vi "Open.vi"(8 "Error In":errorcluster, 9 "StartupConfiguration":string, 11 "reference in":refnum<class "AppConfigJSON.lvclass">) -> (0 "Error Out":errorcluster, 3 "reference out":refnum<class "AppConfigJSON.lvclass">)   [LabVIEW 2021, in "AppConfigJSON.lvclass"]
uses:
  AppConfigJSON.lvclass
  <vilib>/JDP Science/JSONtext/Config Files/Config File.lvclass/Config File.ctl
  1435ef73-8409-4d57-913a-7b04ec8072c7.vi
  aab25018-df5b-4ee7-aaa7-56694cb3da64.vi
  e6364923-a397-4d7b-ac40-c42afb6024f9.vi
  0d2aa625-af8f-4f9d-94fd-328c4132ffee.vi
  <vilib>/TriekselSoft/TracerLibrary/TracerLibrary/Tracer/protected/SendMessage.vi
  <vilib>/TriekselSoft/TracerLibrary/TracerLibrary/Tracer/protected/Timestamp.vi
  0d2aa625-af8f-4f9d-94fd-328c4132ffee.vi/f75db090-0877-4668-94fb-75c2140b1617.vi
  <vilib>/JDP Science/JSONtext/JSON text to Variant.vi
  <vilib>/JDP Science/JSONtext/Variant to JSON Text.vi
  <vilib>/JDP Science/JSONtext/Config Files/Write Config to File.vi
  <vilib>/TriekselSoft/TracerLibrary/TracerLibrary/Tracer/Tracer_Level-Debug.vi
  <vilib>/TriekselSoft/TracerLibrary/TracerLibrary/Tracer/protected/Tracer_ClassAttributes.vi
  <vilib>/JDP Science/JSONtext/LVClass Serializer/JSONtext LVClass Serializer.lvclass
  AppConfigJSON.lvclass/AppConfigJSON.ctl
  <vilib>/JDP Science/JSONtext/Config Files/Config File.lvclass
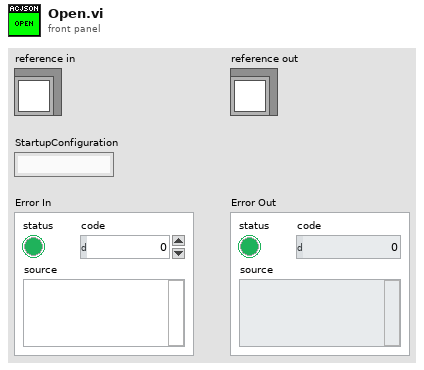
[diagram p1: front panel]
types:
  T1 = typedef "AppConfigJSON.lvclass/ObjectAttributes.ctl" = cluster{"Name":string, "ConfigFilePath":path, "Objects":T2[], "ApplicationBasePath":path, "ObjectName":string}
  T2 = typedef "IApplicationConfiguration.lvclass/ObjectDataDetails.ctl" = cluster{"ObjectName":string, "ObjectType":string, "Interfaces":T3[]}
  T3 = typedef "IApplicationConfiguration.lvclass/ObjectData.ctl" = cluster{"Label":string, "ObjectName":string, "Type":string}
  T4 = cluster{"Objects":cluster{"ObjectName":string, "ObjectType":string, "Interfaces":cluster{"Label":string, "ObjectName":string, "Type":string}[]}[]}
  T5 = cluster{"ObjectName":string, "ObjectType":string, "Interfaces":cluster{"Label":string, "ObjectName":string, "Type":string}[]}[]
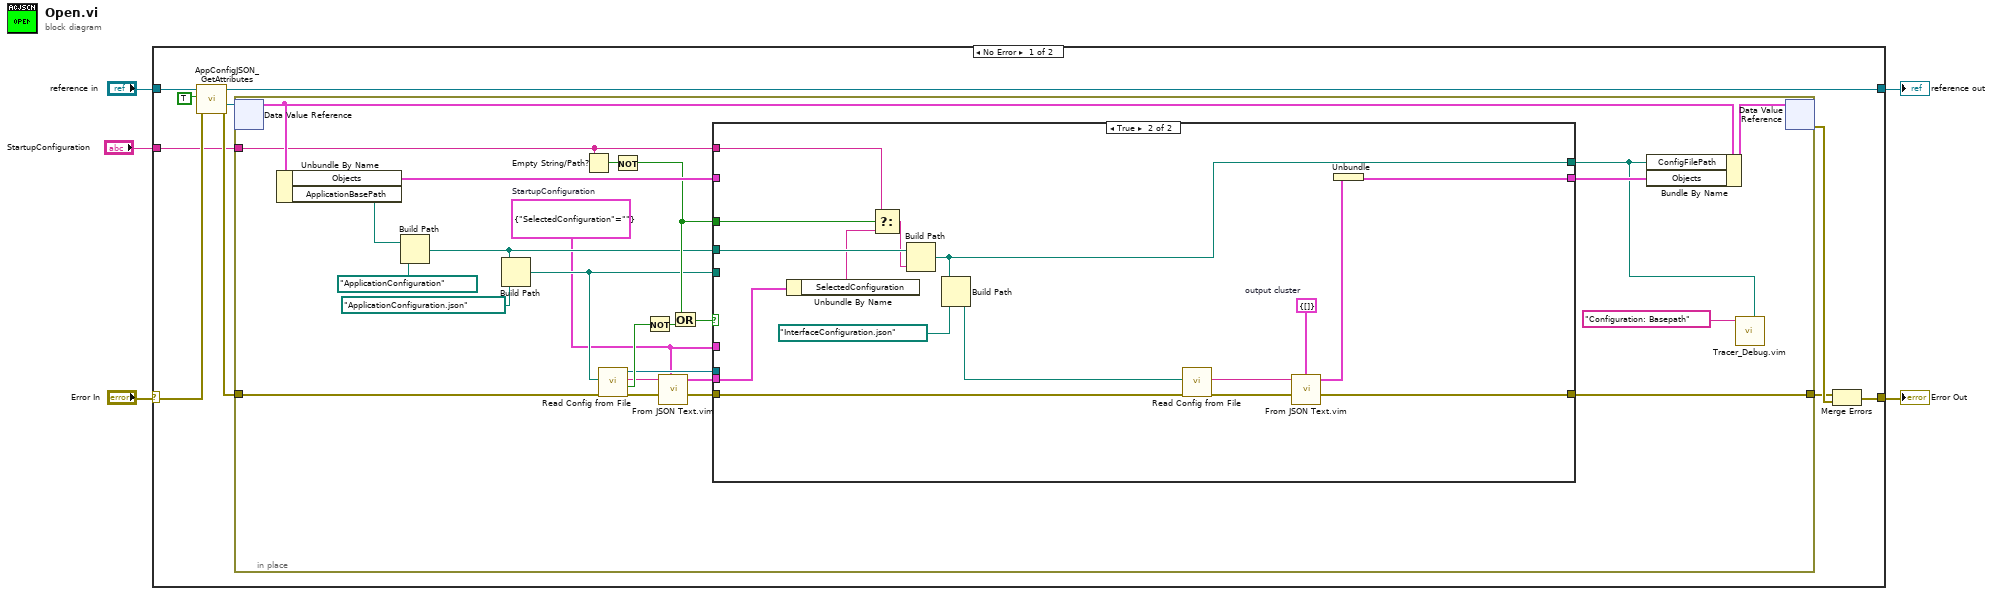
[diagram p0: block diagram]
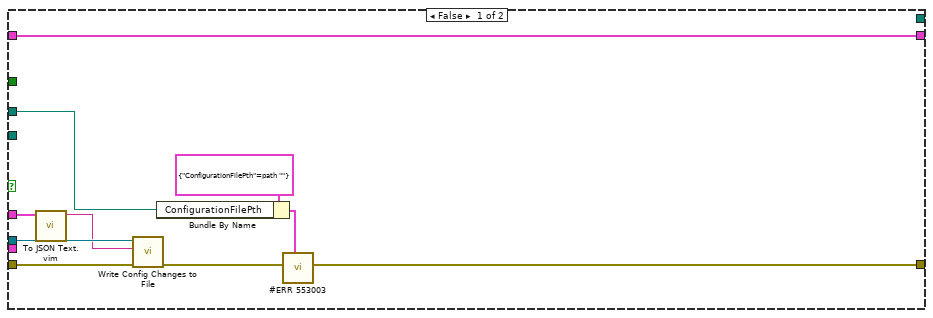
[diagram p2: hidden frame]
diagram:
  n1 = case shown="No Error" "Error In" {
    selector: "Error In" -> [w13 w68]
    tunnel: [w9 w68] -> w4
    tunnel: [w14 w67] -> w2
    tunnel: "reference in" -> [w15 w67]
    tunnel: "StartupConfiguration" -> [w6 _]
    frame No Error {
      n2 = call "AppConfigJSON_GetAttributes.vi"("error in (no error)"=w13, "OnlyGetDvrReference(False)"=TRUE, "reference in"=w15) -> ("error out"=w8:errorcluster, "DataRef"=w10:refnum<data-value>, "reference out"=w14:refnum<class "AppConfigJSON.lvclass">)  [unwired: 5 in, 1 out]
      n3 = in-place {
        in-place-border: w8 -> [w17]
        in-place-border: [w33] -> w7
        in-place-border: w6 -> [w30]
        w16 = cluster{"SelectedConfiguration":string} {"SelectedConfiguration"=""}  # StartupConfiguration
        n4 = in-place-dvr #1(w10) -> (w36:T1)  [unwired: 1 out]
        n5 = Unbundle By Name(w36) -> ("Objects"=w34:T2[], "ApplicationBasePath"=w37:path)
        n6 = Build Path(base path=w37, name or relative path=path "ApplicationConfiguration") -> (appended path=w26:path)
        n7 = Build Path(base path=w26, name or relative path=path "ApplicationConfiguration.json") -> (appended path=w25:path)
        n8 = Empty String/Path?(string/path=w30) -> (empty?=w28:bool)
        n9 = call <vilib>:"Read Config from File.vi"("error in (no error)"=w17, "config file path"=w25) -> ("error out"=w22:errorcluster, "Template Used (file missing or corrupted)"=w24:bool, "<JSON>Config"=w18:string, "Config File"=w19:refnum<class "Config File.lvclass">)  [unwired: 6 in]
        n10 = Not(x=w28) -> (.not. x?=w27:bool)
        n11 = Not(x=w24) -> (.not. x?=w23:bool)
        n12 = call "From JSON Text.vim"("Data Type and Default Value"=w16, "error in (no error)"=w22, "JSON"=w18) -> ("error out"=w21:errorcluster, "Data out"=w20:cluster{"SelectedConfiguration":string})  [unwired: 7 in]
        n13 = Or(x=w27, y=w23) -> (x .or. y?=w29:bool)
        n14 = case shown="True" w29 {
          tunnel: [w50 w53] -> w33
          tunnel: w21 -> [w45 w58]
          tunnel: w26 -> [w48 w66]
          tunnel: w25 -> [_ _]
          tunnel: [w46 w51] -> w35
          tunnel: w34 -> [w46 _]
          tunnel: [_ w60] -> w31
          tunnel: w30 -> [_ w63]
          tunnel: w27 -> [_ w64]
          tunnel: w20 -> [_ w59]
          tunnel: w19 -> [w43 _]
          tunnel: w16 -> [w42 _]
          frame False {
            n15 = call "To JSON Text.vim"("Anything"=w42) -> ("<JSON>"=w41:string)  [unwired: 9 in, 1 out]
            n16 = call <vilib>:"Write Config Changes to File.vi"("error in (no error)"=w45, "New Config"=w41, "Config File in"=w43) -> ("error out"=w44:errorcluster)  [unwired: 5 in, 3 out]
            n17 = Bundle By Name(cluster=cluster{"ConfigurationFilePth":path} {"ConfigurationFilePth"=path ""}, "ConfigurationFilePth"=w48) -> (w47:cluster{"ConfigurationFilePth":path})
            n18 = call "#ERR 553003"("Data"=w47, "error in (no error)"=w44) -> ("error out"=w50:errorcluster)  [unwired: 9 in]
          }
          frame True {
            w56 = T4 {"Objects"=[]}  # output cluster
            n19 = Unbundle By Name(w59) -> ("SelectedConfiguration"=w62:string)
            n20 = Select(t=w63, s=w64, f=w62) -> (s? t:f=w61:string)
            n21 = Build Path(base path=w66, name or relative path=w61) -> (appended path=w60:path)
            n22 = Build Path(base path=w60, name or relative path=path "InterfaceConfiguration.json") -> (appended path=w57:path)
            n23 = call <vilib>:"Read Config from File.vi"("error in (no error)"=w58, "config file path"=w57) -> ("error out"=w54:errorcluster, "<JSON>Config"=w55:string)  [unwired: 6 in, 2 out]
            n24 = call "From JSON Text.vim"("Data Type and Default Value"=w56, "error in (no error)"=w54, "JSON"=w55) -> ("error out"=w53:errorcluster, "Data out"=w52:T4)  [unwired: 7 in]
            n25 = Unbundle(w52) -> ("Objects"=w51:T5)
          }
        }
        n26 = Bundle By Name(cluster=w36, "ConfigFilePath"=w31, "Objects"=w35) -> (w40:T1)
        n27 = call "Tracer_Debug.vim"("Data"=w31, "Text"="Configuration: Basepath") -> ()  [unwired: 9 in, 1 out]
        n28 = in-place-dvr #1(w40) -> (w11:errorcluster)  [unwired: 1 out]
      }
      n29 = Merge Errors(w7, w11) -> (w9:errorcluster)
    }
    frame Error {
    }
  }
  "Error Out" <- w4
  "reference out" <- w2
